vi "Measurement Logic.vi"() -> ()   [LabVIEW 2021, in "Sample.lvlib"]
uses:
  Sample.lvlib
  Measurement Configuration.ctl
  Measurement Results.ctl
  <vilib>/gRPC/Generated APIs/ni/protobuf/types/RPC Messages/ni_protobuf_types_DoubleXYData.ctl
  <vilib>/Plug-In SDKs/Measurements/Measure Call Context/Measure Call Context.lvclass
  <vilib>/gRPC/Generated APIs/ni/protobuf/types/ni.protobuf.types.lvlib
panel:
  out "measure call context out":refnum<class "Measure Call Context.lvclass">
  in  "measure call context in":refnum<class "Measure Call Context.lvclass">
  out "measurement results":T1={"xy data out"={"x_data"=[], "y_data"=[]}, "double array out"=[], "double out"=0.0, "U32 array out"=[0], "U32 out"=0, "U64 array out"=[0], "U64 out"=0, "I32 array out"=[0], "I32 out"=0, "I64 array out"=[0], "I64 out"=0, "bool out"=FALSE, "string out"="Empty", "u32 color ring out"=0, "u32 animal enum out"=enum."Rabbit"} {"u32 color ring out" items=["Red", "Green", "Blue"]}
  in  "measurement configuration":T3={"double array in"=[], "double in"=1.2, "U32 array in"=[], "U32 in"=0, "U64 array in"=[], "U64 in"=0, "I32 array in"=[], "I32 in"=0, "I64 array in"=[], "I64 in"=0, "bool in"=TRUE, "string in"="Lorem ipsum dolor sit", "u32 color ring in"=1, "u32 animal enum in"=enum."Gopher"} {"u32 color ring in" items=["Red", "Green", "Blue"]}
  out "error out":errorcluster
  in  "error in":errorcluster
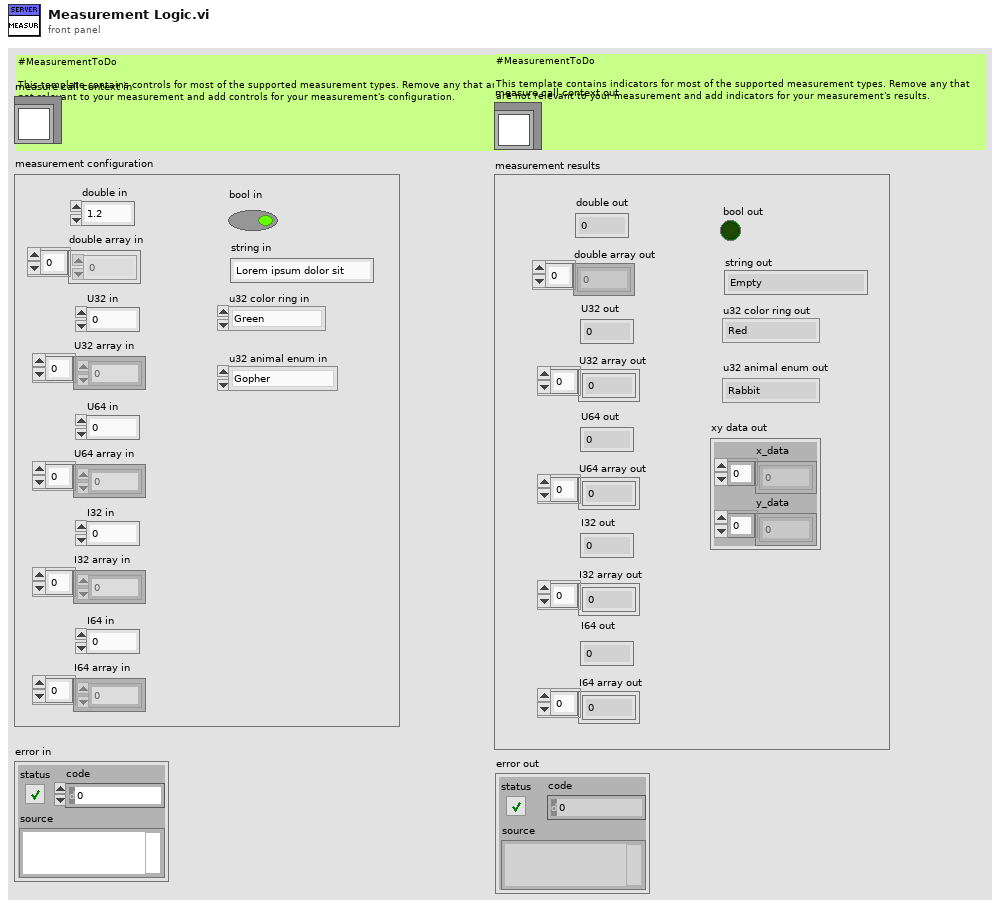
[diagram p1: front panel]
types:
  T1 = typedef "Sample.lvlib/Measurement Results.ctl" = cluster{"xy data out":T2, "double array out":dbl[], "double out":dbl, "U32 array out":u32[], "U32 out":u32, "U64 array out":u64[], "U64 out":u64, "I32 array out":i32[], "I32 out":i32, "I64 array out":i64[], "I64 out":i64, "bool out":bool, "string out":string, "u32 color ring out":u32, "u32 animal enum out":enum32{"Rabbit", "Gopher", "Badger"}}
  T2 = typedef "ni.protobuf.types.lvlib/ni_protobuf_types_DoubleXYData.ctl" = cluster{"x_data":dbl[], "y_data":dbl[]}
  T3 = typedef "Sample.lvlib/Measurement Configuration.ctl" = cluster{"double array in":dbl[], "double in":dbl, "U32 array in":u32[], "U32 in":u32, "U64 array in":u64[], "U64 in":u64, "I32 array in":i32[], "I32 in":i32, "I64 array in":i64[], "I64 in":i64, "bool in":bool, "string in":string, "u32 color ring in":u32, "u32 animal enum in":enum32{"Rabbit", "Gopher", "Badger"}}
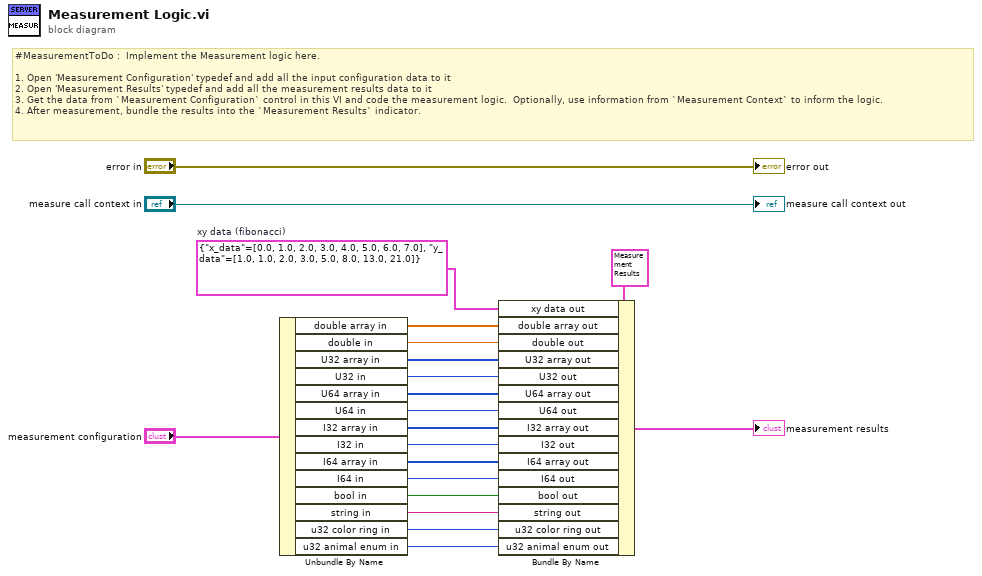
[diagram p0: block diagram]
diagram:
  w1 = T2 {"x_data"=[0.0, 1.0, 2.0, 3.0, 4.0, 5.0, 6.0, 7.0], "y_data"=[1.0, 1.0, 2.0, 3.0, 5.0, 8.0, 13.0, 21.0]}  # xy data (fibonacci)
  # "#MeasurementToDo :  Implement the Measurement logic here.\n\n1. Open 'Measurement Configuration' typedef and add all the input configuration data to it\n2. Open 'Measurement Results' typedef and add all the measurement results data to it\n3. Get the data from `Measurement Configuration` control in this VI and code the measurement logic.  Optionally, use information from `Measurement Context` to inform the logic.\n4. After measurement, bundle the results into the `Measurement Results` indicator."
  n1 = Unbundle By Name("measurement configuration") -> ("double array in"=w15:dbl[], "double in"=w14:dbl, "U32 array in"=w13:u32[], "U32 in"=w12:u32, "U64 array in"=w11:u64[], "U64 in"=w10:u64, "I32 array in"=w9:i32[], "I32 in"=w8:i32, "I64 array in"=w7:i64[], "I64 in"=w6:i64, "bool in"=w5:bool, "string in"=w4:string, "u32 color ring in"=w3:u32, "u32 animal enum in"=w2:enum32{"Rabbit", "Gopher", "Badger"})
  n2 = Bundle By Name(cluster=T1 {"xy data out"={"x_data"=[], "y_data"=[]}, "double array out"=[], "double out"=0.0, "U32 array out"=[0], "U32 out"=0, "U64 array out"=[0], "U64 out"=0, "I32 array out"=[0], "I32 out"=0, "I64 array out"=[0], "I64 out"=0, "bool out"=FALSE, "string out"="Empty", "u32 color ring out"=0, "u32 animal enum out"=enum."Rabbit"} ("Measurement Results"), "xy data out"=w1, "double array out"=w15, "double out"=w14, "U32 array out"=w13, "U32 out"=w12, "U64 array out"=w11, "U64 out"=w10, "I32 array out"=w9, "I32 out"=w8, "I64 array out"=w7, "I64 out"=w6, "bool out"=w5, "string out"=w4, "u32 color ring out"=w3, "u32 animal enum out"=w2) -> (→"measurement results":T1)
  "error out" <- "error in"
  "measure call context out" <- "measure call context in"
